vi "MicroStruct-XY - Learn.vi"() -> ()   [LabVIEW 2014]
doc: "Newport Motion Controler\nThis program make lines structure\n\nAndré Romero - 2020\nandretec@ifsc.usp.br"
uses:
  <vilib>/Platform/TimedLoop/XDataNode/timing_clust.ctl
  <vilib>/Platform/TimedLoop/XDataNode/nitl_modes.ctl
  <vilib>/Platform/TimedLoop/XDataNode/wakeup.ctl
  <vilib>/Platform/TimedLoop/XDataNode/XDataNode.xnode
  <userlib>/Newport ESP301/Newport ESP301.lvlib
  <vilib>/Platform/TimedLoop/XDataNode/XDNodeRunTimeDep.lvlib
panel:
  out "XY Graph":cluster{dbl[], dbl[]}(graph)={[0.0, 0.0, 0.0345, 0.108, 0.2205, 0.3735, 0.564, 0.7665, 0.964, 1.0005, 1.0, 0.9995, 0.9995, 0.9815, 0.9225, 0.8235, 0.686, 0.505, 0.308, 0.108, -0.002, 0.0, 0.0005, 0.0, 0.012, 0.066, 0.1575, 0.2915, 0.465, 0.6645, 0.866, 1.0025, 1.0, 1.0, 0.9995, 0.9965, 0.9565, 0.8775, 0.7585, 0.6, 0.4055, 0.204, 0.006, -0.0005, 0.0005, 0.0, 0.0005, 0.0345, 0.108, 0.2215, 0.375, 0.566, 0.7675, 0.9685, 1.001, 1.0, 1.0, 0.9995, 0.9855, 0.9315, 0.8375, 0.7035, 0.5295, 0.331, 0.1305, -0.0025, 0.0, 0.0005, 0.0, 0.009, 0.0585, 0.148, 0.2765, 0.4475, 0.645, 0.8435, 1.003, 1.0005, 1.0, 0.9995, 0.999, 0.9625, 0.887, 0.773, 0.6175, 0.4265, 0.225, 0.028, -0.0005, 0.0005, 0.0, 0.0005, 0.031, 0.1025, 0.2125, 0.364, 0.55, 0.751, 0.9525, 1.001, 1.0, 1.0, 0.9995, 0.986, 0.9315, 0.8385, 0.705, 0.531, 0.3315, 0.1305, -0.002, 0.0, 0.0005, 0.0, 0.0085, 0.057, 0.146, 0.2735, 0.44, 0.6395, 0.8415, 1.003, 1.0, 1.0, 1.0, 0.9995, 0.9645, 0.891, 0.7775, 0.6255, 0.4355, 0.2345, 0.033, -0.0005, 0.0005, 0.0, 0.0, 0.0185, 0.0775, 0.1765, 0.3145, 0.4925, 0.6925, 0.895, 1.002, 1.0, 1.0, 0.9995, 0.9865, 0.933, 0.839, 0.7055, 0.535, 0.333, 0.1325, -0.0025, 0.0, 0.0005, 0.0, 0.0025, 0.043, 0.1225, 0.2425, 0.4015, 0.5945, 0.795, 0.9955, 1.0005, 1.0, 1.0, 0.9995, 0.965, 0.8915, 0.7775, 0.625, 0.4335, 0.235, 0.035, -0.0005, 0.0005, 0.0, 0.0, 0.0185, 0.078, 0.176, 0.3155, 0.4925, 0.693, 0.892, 1.002, 1.0, 1.0, 0.9995, 0.9865, 0.933, 0.8405, 0.706, 0.5345, 0.3325, 0.1335, -0.0025, 0.0, 0.0005, 0.0, 0.002, 0.043, 0.1225, 0.2415, 0.401, 0.594, 0.7955, 0.9945, 1.0005, 1.0, 0.9995, 0.9995, 0.9655, 0.891, 0.7775, 0.623, 0.431, 0.233, 0.032, 0.0, 0.0005, 0.0, 0.0], [0.0, 0.0, 0.0, 0.0, 0.0, 0.0, 0.0, 0.0, 0.0, 0.0, 0.021, 0.0825, 0.1015, 0.101, 0.1005, 0.1, 0.1, 0.1, 0.1, 0.1, 0.1, 0.104, 0.158, 0.2015, 0.2015, 0.2005, 0.2, 0.2, 0.2, 0.2, 0.2, 0.2, 0.2, 0.2425, 0.3015, 0.3015, 0.301, 0.3005, 0.3, 0.3, 0.3, 0.3, 0.3, 0.3, 0.328, 0.3975, 0.4015, 0.401, 0.4005, 0.4, 0.4, 0.4, 0.4, 0.4, 0.4, 0.411, 0.468, 0.5015, 0.501, 0.5005, 0.5, 0.5, 0.5, 0.5, 0.5, 0.5, 0.504, 0.557, 0.6015, 0.601, 0.6005, 0.6, 0.6, 0.6, 0.6, 0.6, 0.6, 0.6, 0.6365, 0.7015, 0.7015, 0.701, 0.7, 0.7, 0.7, 0.7, 0.7, 0.7, 0.7, 0.7275, 0.7955, 0.8015, 0.801, 0.8005, 0.8, 0.8, 0.8, 0.8, 0.8, 0.8, 0.8105, 0.868, 0.902, 0.9015, 0.9, 0.9, 0.9, 0.9, 0.9, 0.9, 0.9, 0.9005, 0.9485, 1.0015, 1.0015, 1.0005, 1.0, 1.0, 1.0, 0.9995, 0.9995, 1.0, 1.0, 1.0345, 1.1015, 1.1015, 1.101, 1.1, 1.1, 1.1, 1.1, 1.1, 1.1, 1.1, 1.128, 1.1865, 1.2015, 1.201, 1.2, 1.2, 1.2, 1.1995, 1.2, 1.2, 1.2, 1.207, 1.259, 1.3015, 1.3015, 1.3005, 1.3, 1.3, 1.3, 1.3, 1.3, 1.3, 1.3, 1.343, 1.4015, 1.4015, 1.4005, 1.4, 1.4, 1.4, 1.4, 1.3995, 1.3995, 1.4, 1.429, 1.4985, 1.5015, 1.5005, 1.5, 1.5, 1.5, 1.5, 1.5, 1.5, 1.5, 1.5175, 1.578, 1.6015, 1.601, 1.6005, 1.6, 1.6, 1.6, 1.6, 1.6, 1.6, 1.605, 1.659, 1.7015, 1.701, 1.7005, 1.7, 1.7, 1.7, 1.7, 1.7, 1.7, 1.7, 1.7425, 1.802, 1.8015, 1.8005, 1.8, 1.8, 1.8, 1.8, 1.8, 1.8, 1.8, 1.8295, 1.8995, 1.9015, 1.9005, 1.9, 1.9, 1.9, 1.9, 1.9, 1.8995, 1.8995, 1.918, 1.979, 2.002]}
  in  "N Cycles":i32=10 min=1
  in  "Acceleration (0 units/s²)":dbl=1.0 min=0.0 format="%#.4g"
  in  "Velocity (units/s)":dbl=1.0 min=0.0 format="%#.4g"
  in  "d (mm)":dbl=0.1
  in  "L (mm)":dbl=1.0
  out "X Position (mm)":dbl format="%.6g"
  out "Y Position (mm)":dbl=2.002 format="%.6g"
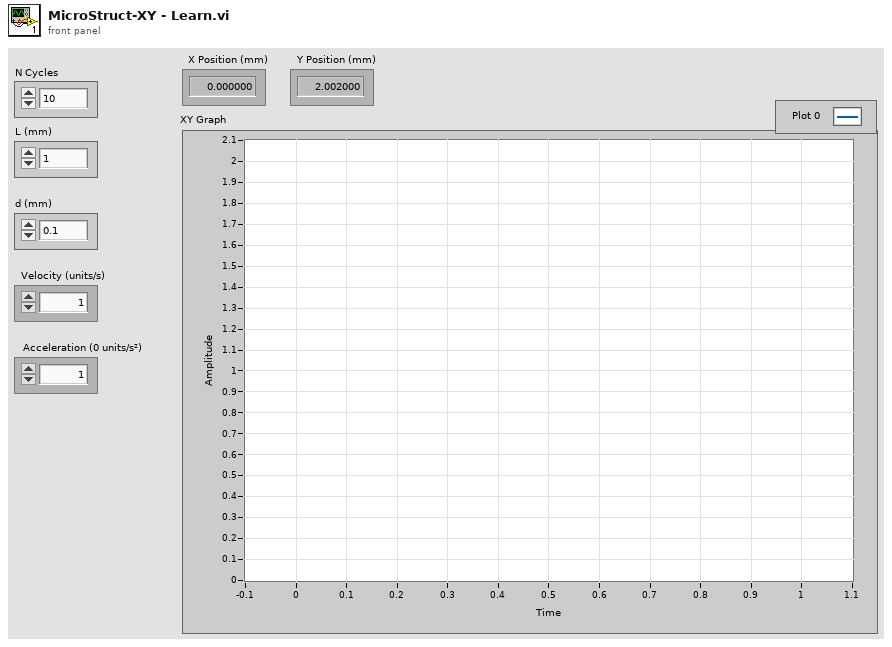
[diagram p1: front panel]
types:
  T1 = typedef "XDNodeRunTimeDep.lvlib/timing_clust.ctl" = cluster{"Expected End [f-1]":u64, "Actual End [f-1]":u64, "Finished Late? [f-1]":bool, "Expected End [i-1]":u64, "Actual End [i-1]":u64, "Finished Late? [i-1]":bool, "Expected Start [i]":u64, "Actual Start [i]":u64, "Expected Start [f]":u64, "Actual Start [f]":u64, "Source Name":string, "Structure Name":string, "Period":i64, "Deadline":i64, "Offset":i64, "Start":i64, "Priority":i32, "Timeout":i32, "Mode":T2, "Wakeup Reason":T3, "Error":errorcluster, "Source Type":string, "Secondary Source Type":string, "Global End Time":u64, "Global Start Time":u64, "Frame Duration":u64, "Iteration Duration":u64, "Assigned CPU":i32, "I/O Scan Engine Mode":u32}
  T2 = typedef "XDNodeRunTimeDep.lvlib/nitl_modes.ctl" = enum32{"No Change", "Process missed periods, maintain original phase", "Discard missed periods, maintain original phase", "Process missed periods, ignore original phase", "Discard missed periods, ignore original phase"}
  T3 = typedef "XDNodeRunTimeDep.lvlib/wakeup.ctl" = enum32{"Normal", "Aborted", "Asynchronous wakeup", "Timing source error", "Timed loop error", "Timeout"}
  T4 = cluster{"Axis1 moving":bool, "Axis2 moving":bool, "Axis3 moving":bool, "Axis4 moving":bool, "Motor Power of at least one axis":bool, "Reserved":bool, "Reserved":bool, "Reserved":bool, "Axis5 moving 2":bool, "Axis6 moving 2":bool, "Reserved":bool, "Reserved":bool, "Motor Power of at least one axis":bool, "Reserved":bool, "Reserved":bool, "Reserved":bool}
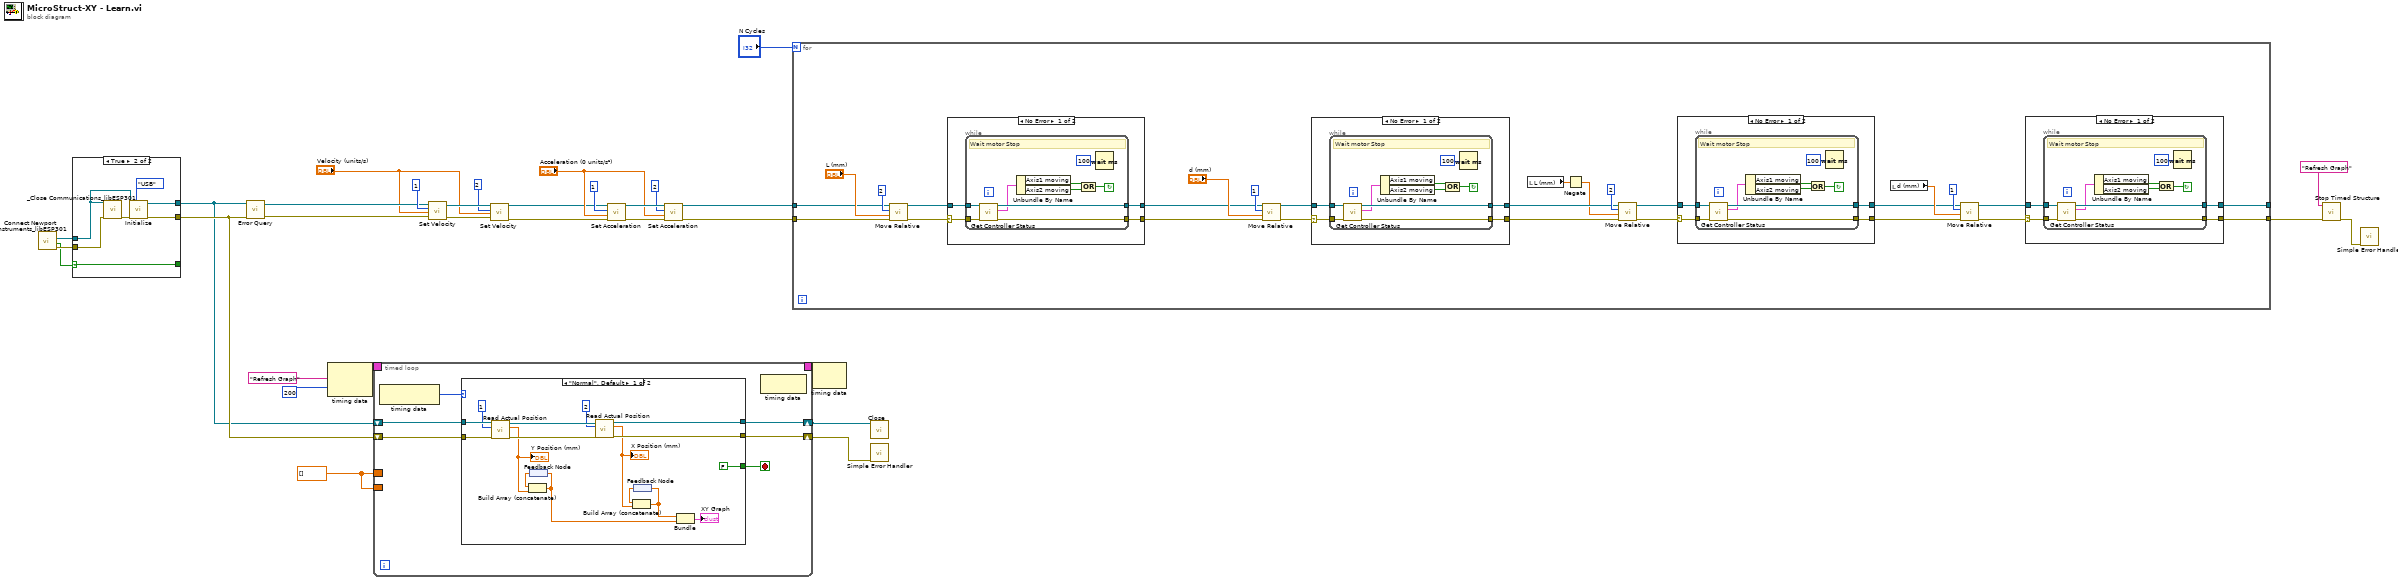
[diagram p0: block diagram]
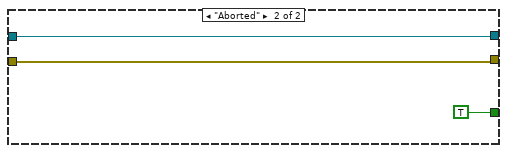
[diagram p6: hidden frame]
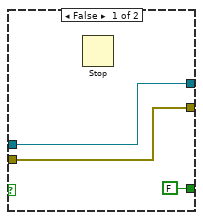
[diagram p7: hidden frame]
diagram:
  w3 = dbl[] []
  n1 = call <userlib>:"Connect Newport Instruments_libESP301.vi"() -> ("error (duplicate)"=w32:errorcluster, "Connected"=w26:bool, "VISA resource name (duplicate)"=w31:refnum<visa-resource-name>)  [unwired: 7 in, 2 out]
  n2 = case shown="True" w26 {
    selector: w26 -> [_ w36]
    tunnel: w32 -> [w33 w40]
    tunnel: w31 -> [w34 w39]
    tunnel: [w33 w38] -> w30
    tunnel: [w34 w37] -> w29
    tunnel: [FALSE w36] -> _
    frame False {
      n3 = Stop() -> ()  [unwired: 1 in]
    }
    frame True {
      n4 = call <userlib>:"_Close Communications_libESP301.vi"("Instrument Channel"=w39, "error in (no error)"=w40) -> ("error out"=w42:errorcluster)  [unwired: 13 in]
      n5 = call <userlib>:"Initialize.vi"("VISA resource name"=w39, "error in (no error)"=w42, "Serial Link (RS232)"=enum16{"RS232", "USB"}."USB") -> ("VISA resource name out"=w37:refnum<visa-resource-name>, "error out"=w38:errorcluster)  [unwired: 6 in]
    }
  }
  n6 = call <userlib>:"Error Query.vi"("error in (no error)"=w30, "VISA resource name"=w29) -> ("error out"=w19:errorcluster, "VISA resource name out"=w17:refnum<visa-resource-name>)  [unwired: 2 in, 2 out]
  n7 = node-c288("Refresh Graph" ("Structure Name"), i64 200 ("Period")) -> (w25:T1)
  n8 = timed-loop {
    timing: w25 -> [_]
    timing-out: [_] -> w24
    shift-right: [w46] -> w28
    shift-left: w29 -> [w48]
    shift-right: [w45] -> w27
    shift-left: w30 -> [w47]
    border: w3 -> [_]
    border: w3 -> [_]
    stop <- w43 stop-if-true
    n9 = node-c288() -> (w44:T3)  [unwired: 1 in]
    n10 = case shown="\"Normal\", Default" w44 {
      tunnel: w48 -> [w64 w66]
      tunnel: w47 -> [w63 w65]
      tunnel: [w60 w66] -> w46
      tunnel: [w59 w65] -> w45
      tunnel: [FALSE TRUE] -> w43
      frame "Normal", Default {
        n11 = call <userlib>:"Read Actual Position.vi"("error in (no error)"=w63, "Axis (1)"=1, "VISA resource name"=w64) -> ("error out"=w61:errorcluster, "Position (units)"=w52:dbl, "VISA resource name out"=w62:refnum<visa-resource-name>)  [unwired: 2 in]
        "Y Position (mm)" <- w52
        n12 = feedback #1() -> (w55:dbl[])
        n13 = Build Array (concatenate)(w55, w52) -> (w50:dbl[])
        n14 = feedback-in #1(w50) -> ()
        n15 = call <userlib>:"Read Actual Position.vi"("error in (no error)"=w61, "Axis (1)"=2, "VISA resource name"=w62) -> ("error out"=w59:errorcluster, "Position (units)"=w53:dbl, "VISA resource name out"=w60:refnum<visa-resource-name>)  [unwired: 2 in]
        "X Position (mm)" <- w53
        n16 = feedback #2() -> (w54:dbl[])
        n17 = Build Array (concatenate)(w54, w53) -> (w51:dbl[])
        n18 = feedback-in #2(w51) -> ()
        n19 = Bundle(w51, w50) -> (→"XY Graph":cluster{dbl[], dbl[]})  [unwired: 1 in]
      }
      frame "Aborted" {
      }
    }
    n20 = node-c288() -> ()  [unwired: 1 in, 1 out]
  }
  n21 = call <userlib>:"Set Velocity.vi"("error in (no error)"=w19, "Velocity (units/s)"="Velocity (units/s)", "Axis (1)"=1, "VISA resource name"=w17) -> ("error out"=w21:errorcluster, "VISA resource name out"=w22:refnum<visa-resource-name>)  [unwired: 2 in]
  n22 = call <userlib>:"Set Velocity.vi"("error in (no error)"=w21, "Velocity (units/s)"="Velocity (units/s)", "Axis (1)"=2, "VISA resource name"=w22) -> ("error out"=w9:errorcluster, "VISA resource name out"=w10:refnum<visa-resource-name>)  [unwired: 2 in]
  n23 = call <userlib>:"Set Acceleration.vi"("error in (no error)"=w9, "Acceleration (0 units/s²)"="Acceleration (0 units/s²)", "Axis (1)"=1, "VISA resource name"=w10) -> ("error out"=w14:errorcluster, "VISA resource name out"=w15:refnum<visa-resource-name>)  [unwired: 2 in]
  n24 = call <userlib>:"Set Acceleration.vi"("error in (no error)"=w14, "Acceleration (0 units/s²)"="Acceleration (0 units/s²)", "Axis (1)"=2, "VISA resource name"=w15) -> ("error out"=w7:errorcluster, "VISA resource name out"=w8:refnum<visa-resource-name>)  [unwired: 2 in]
  n25 = for {
    N: "N Cycles" -> [_]
    tunnel: w8 -> [w74]
    tunnel: w7 -> [w73]
    tunnel: [w72] -> _
    tunnel: [w71] -> w2
    n26 = call <userlib>:"Move Relative.vi"("error in (no error)"=w73, "Position (0 units)"="L (mm)", "Axis (1)"=2, "VISA resource name"=w74) -> ("error out"=w95:errorcluster, "VISA resource name out"=w96:refnum<visa-resource-name>)  [unwired: 2 in]
    n27 = case shown="No Error" w95 {
      selector: w95 -> [w146 w156]
      tunnel: w96 -> [w145 w157]
      tunnel: [w144 w157] -> w91
      tunnel: [w143 w156] -> w90
      frame No Error {
        n28 = while {
          tunnel: [w154] -> w144
          tunnel: w146 -> [w155]
          tunnel: [w153] -> w143
          tunnel: w145 -> [w147]
          stop <- w149 continue-if-true
          # "Wait motor Stop"
          n29 = call <userlib>:"Get Controller Status.vi"("error in (no error)"=w155, "VISA resource name"=w147) -> ("error out"=w153:errorcluster, "Controller Status"=w152:T4, "VISA resource name out"=w154:refnum<visa-resource-name>)  [unwired: 2 in, 1 out]
          n30 = Unbundle By Name(w152) -> ("Axis1 moving"=w151:bool, "Axis2 moving"=w150:bool)
          n31 = Compound Arithmetic op=OR(w151, w150) -> (w149:bool)
          n32 = Wait (ms)(milliseconds to wait=u32 100) -> ()  [unwired: 1 out]
        }
      }
      frame Error {
      }
    }
    n33 = call <userlib>:"Move Relative.vi"("error in (no error)"=w90, "Position (0 units)"="d (mm)", "Axis (1)"=1, "VISA resource name"=w91) -> ("error out"=w88:errorcluster, "VISA resource name out"=w89:refnum<visa-resource-name>)  [unwired: 2 in]
    n34 = case shown="No Error" w88 {
      selector: w88 -> [w131 w141]
      tunnel: w89 -> [w130 w142]
      tunnel: [w129 w142] -> w83
      tunnel: [w128 w141] -> w82
      frame No Error {
        n35 = while {
          tunnel: [w139] -> w129
          tunnel: w131 -> [w140]
          tunnel: [w138] -> w128
          tunnel: w130 -> [w132]
          stop <- w134 continue-if-true
          # "Wait motor Stop"
          n36 = call <userlib>:"Get Controller Status.vi"("error in (no error)"=w140, "VISA resource name"=w132) -> ("error out"=w138:errorcluster, "Controller Status"=w137:T4, "VISA resource name out"=w139:refnum<visa-resource-name>)  [unwired: 2 in, 1 out]
          n37 = Unbundle By Name(w137) -> ("Axis1 moving"=w136:bool, "Axis2 moving"=w135:bool)
          n38 = Compound Arithmetic op=OR(w136, w135) -> (w134:bool)
          n39 = Wait (ms)(milliseconds to wait=u32 100) -> ()  [unwired: 1 out]
        }
      }
      frame Error {
      }
    }
    n40 = local read "L (mm)"() -> (w84:dbl)
    n41 = Negate(x=w84) -> (-x=w75:dbl)
    n42 = call <userlib>:"Move Relative.vi"("error in (no error)"=w82, "Position (0 units)"=w75, "Axis (1)"=2, "VISA resource name"=w83) -> ("error out"=w85:errorcluster, "VISA resource name out"=w86:refnum<visa-resource-name>)  [unwired: 2 in]
    n43 = case shown="No Error" w85 {
      selector: w85 -> [w116 w126]
      tunnel: w86 -> [w115 w127]
      tunnel: [w114 w127] -> w76
      tunnel: [w113 w126] -> w78
      frame No Error {
        n44 = while {
          tunnel: [w124] -> w114
          tunnel: w116 -> [w125]
          tunnel: [w123] -> w113
          tunnel: w115 -> [w117]
          stop <- w119 continue-if-true
          # "Wait motor Stop"
          n45 = call <userlib>:"Get Controller Status.vi"("error in (no error)"=w125, "VISA resource name"=w117) -> ("error out"=w123:errorcluster, "Controller Status"=w122:T4, "VISA resource name out"=w124:refnum<visa-resource-name>)  [unwired: 2 in, 1 out]
          n46 = Unbundle By Name(w122) -> ("Axis1 moving"=w121:bool, "Axis2 moving"=w120:bool)
          n47 = Compound Arithmetic op=OR(w121, w120) -> (w119:bool)
          n48 = Wait (ms)(milliseconds to wait=u32 100) -> ()  [unwired: 1 out]
        }
      }
      frame Error {
      }
    }
    n49 = local read "d (mm)"() -> (w77:dbl)
    n50 = call <userlib>:"Move Relative.vi"("error in (no error)"=w78, "Position (0 units)"=w77, "Axis (1)"=1, "VISA resource name"=w76) -> ("error out"=w79:errorcluster, "VISA resource name out"=w80:refnum<visa-resource-name>)  [unwired: 2 in]
    n51 = case shown="No Error" w79 {
      selector: w79 -> [w101 w111]
      tunnel: w80 -> [w100 w112]
      tunnel: [w99 w112] -> w72
      tunnel: [w98 w111] -> w71
      frame No Error {
        n52 = while {
          tunnel: [w109] -> w99
          tunnel: w101 -> [w110]
          tunnel: [w108] -> w98
          tunnel: w100 -> [w102]
          stop <- w104 continue-if-true
          # "Wait motor Stop"
          n53 = call <userlib>:"Get Controller Status.vi"("error in (no error)"=w110, "VISA resource name"=w102) -> ("error out"=w108:errorcluster, "Controller Status"=w107:T4, "VISA resource name out"=w109:refnum<visa-resource-name>)  [unwired: 2 in, 1 out]
          n54 = Unbundle By Name(w107) -> ("Axis1 moving"=w106:bool, "Axis2 moving"=w105:bool)
          n55 = Compound Arithmetic op=OR(w106, w105) -> (w104:bool)
          n56 = Wait (ms)(milliseconds to wait=u32 100) -> ()  [unwired: 1 out]
        }
      }
      frame Error {
      }
    }
  }
  n57 = node-c288(w24) -> ()  [unwired: 1 out]
  n58 = call <userlib>:"Close.vi"("VISA resource name"=w28) -> ()  [unwired: 10 in, 1 out]
  n59 = call <vilib>:"Simple Error Handler.vi"("error in (no error)"=w27) -> ()  [unwired: 1 in, 8 out]
  n60 = call <vilib>:"Stop Timed Structure.vi"("error in (no error)"=w2, "name"="Refresh Graph" ("Structure Name")) -> ("error out"=w1:errorcluster)  [unwired: 9 in]
  n61 = call <vilib>:"Simple Error Handler.vi"("error in (no error)"=w1) -> ()  [unwired: 4 in, 5 out]
